vi "Array2String.vi"(10 "Plate":string, 11 "Array_Input":i8[](array[numeric])) -> (3 "String_Out":string)   [LabVIEW 2020]
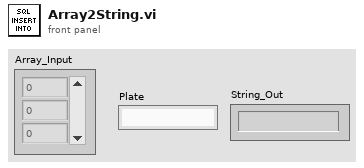
[diagram p1: front panel]
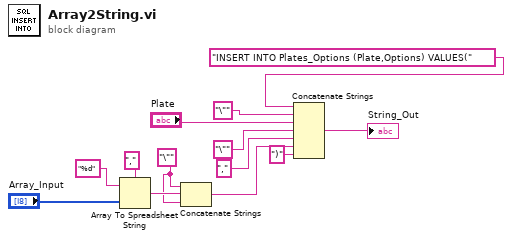
[diagram p0: block diagram]
diagram:
  w10 = "\""
  n1 = Array To Spreadsheet String(delimiter (Tab)=",", array="Array_Input", 3:"%d" ("format string")) -> (spreadsheet string=w11:string)
  n2 = Concatenate Strings(w10, w11, w10) -> (w2:string)
  n3 = Concatenate Strings("INSERT INTO Plates_Options (Plate,Options) VALUES(", "\"", "Plate", "\"", "," ("delimiter (Tab)"), w2, ")" ("string")) -> (→"String_Out":string)
